vi "Write in logger.vi"(3 "error in":errorcluster, 4 "String in":string, 5 "logger refnum":refnum<file>) -> (0 "error out":errorcluster, 2 "refnum out":refnum<file>)   [LabVIEW 2017]
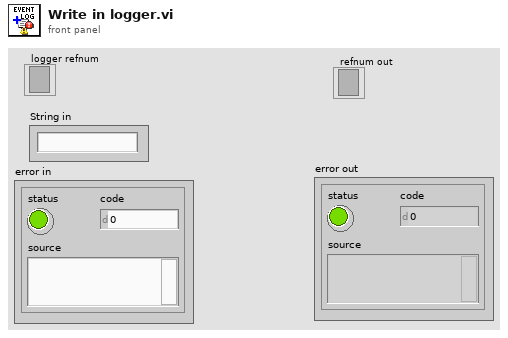
[diagram p1: front panel]
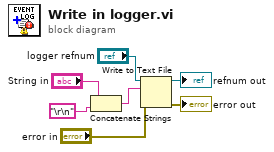
[diagram p0: block diagram]
diagram:
  n1 = Concatenate Strings("String in", "\r\n") -> (w7:string)
  n2 = Write to Text File(file (use dialog)="logger refnum", text=w7, error in="error in") -> (refnum out=→"refnum out":refnum<file>, error out=→"error out":errorcluster)  [unwired: 1 in, 1 out]
